vi "Key.vi"(11 "Identity in":refnum<class "Identity.lvclass">) -> (2 "Key":string)   [LabVIEW 2020, in "Volatus.lvlib" / "Identity.lvclass"]
uses:
  Identity.lvclass
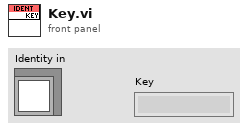
[diagram p1: front panel]
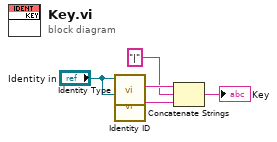
[diagram p0: block diagram]
diagram:
  n1 = call-dynamic "Identity Type.vi"("Identity in"="Identity in") -> ("Type"=w4:string)  [unwired: 10 in]
  n2 = call-dynamic "Identity ID.vi"("Identity in"="Identity in") -> ("ID"=w3:string)  [unwired: 10 in]
  n3 = Concatenate Strings(w4, "|" ("string"), w3) -> (→"Key":string)
